vi "LVClass_WavefrontCorrectorSet Get Parameter Int Default Value.vi"(0 "WavefrontCorrectorSet in":refnum<class "WavefrontCorrectorSet.lvclass">, 5 "parameter_name":string, 11 "error in (no error)":errorcluster) -> (4 "WavefrontCorrectorSet out":refnum<class "WavefrontCorrectorSet.lvclass">, 6 "Default value":i32, 15 "error out":errorcluster)   [LabVIEW 2020, in "WavefrontCorrectorSet.lvclass"]
doc: "WavefrontCorrector parameter default value getter for parameter of type\ninteger.\n\n--------------------------------------------------------------------------------\n\n<B>wavefrontcorrector_setIn </B> : WavefrontCorrectorSet object.\n<B>wavefrontcorrector_setOut </B> : WavefrontCorrectorSet object.\n<B>parameter_name </B> : Parameter name.\n<B>default_value </B> : Parameter default value.\n<B>ErrorIn </B> : Error\n<B>ErrorOut </B> : Error\n\n--------------------------------------------------------------------------------"
uses:
  WavefrontCorrectorSet.lvclass
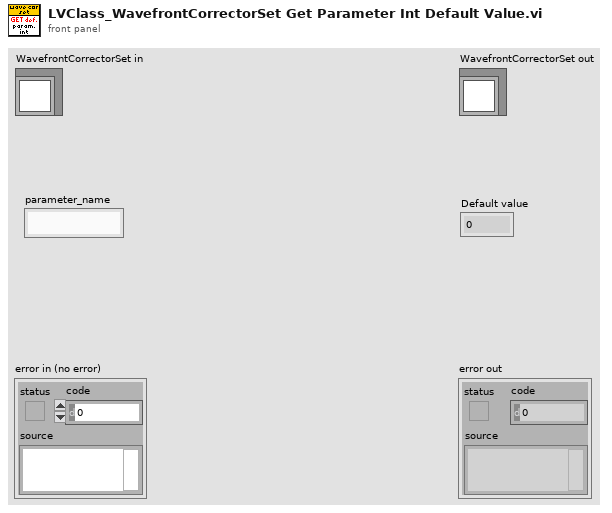
[diagram p1: front panel]
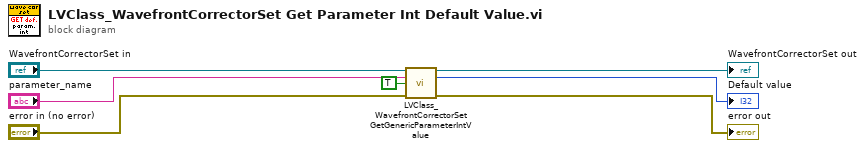
[diagram p0: block diagram]
diagram:
  n1 = call "LVClass_WavefrontCorrectorSet GetGenericParameterIntValue.vi"("WavefrontCorrectorSet in"="WavefrontCorrectorSet in", "parameter_name"="parameter_name", "DefaultFactorySet"=TRUE, "error in (no error)"="error in (no error)") -> ("WavefrontCorrectorSet out"=→"WavefrontCorrectorSet out":refnum<class "WavefrontCorrectorSet.lvclass">, "Value"=→"Default value":i32, "error out"=→"error out":errorcluster)  [unwired: 9 in]
